vi "Set QMH Payload.vi"(8 "error in (no error)":errorcluster, 9 "Data":variant, 10 "State":enum16{""}(ring), 11 "IMessagePayload in":refnum<class "IMessagePayload.lvclass">) -> (0 "error out":errorcluster, 3 "IMessagePayload":refnum<class "IMessagePayload.lvclass">)   [LabVIEW 2016, in "QMHMessagePayload.lvclass"]
uses:
  QMHMessagePayload.lvclass
  IMessagePayload/IMessagePayload.lvclass
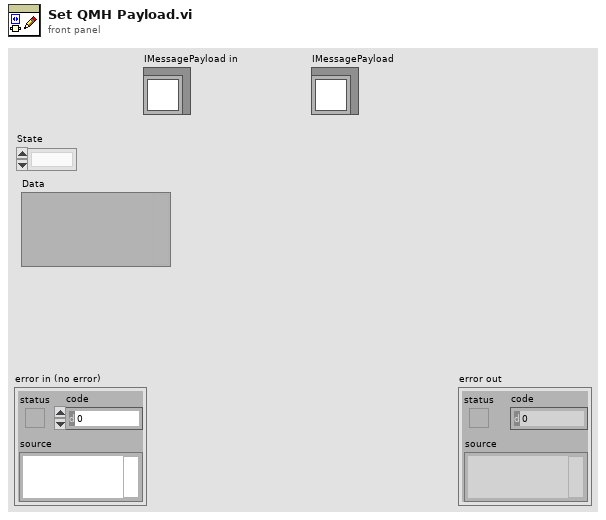
[diagram p1: front panel]
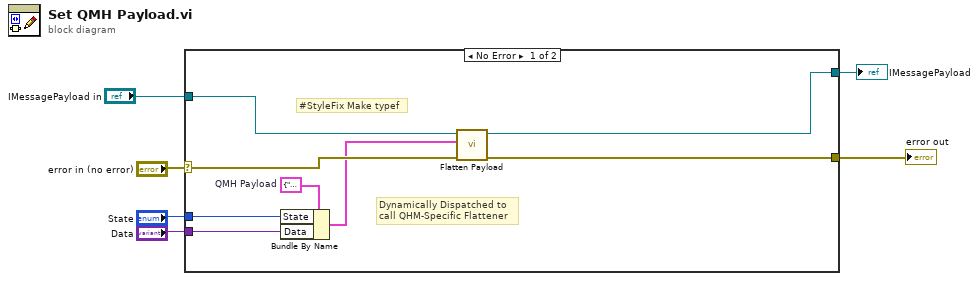
[diagram p0: block diagram]
diagram:
  n1 = case shown="No Error" "error in (no error)" {
    selector: "error in (no error)" -> [w14 w15]
    tunnel: [w13 w15] -> w5
    tunnel: "IMessagePayload in" -> [w12 _]
    tunnel: [w11 _] -> w3
    tunnel: "State" -> [w8 _]
    tunnel: "Data" -> [w7 _]
    frame No Error {
      w10 = cluster{"State":enum16{""}, "Data":variant} {"State"=enum."", "Data"=variant}  # QMH Payload
      # "#StyleFix Make typef"
      # "Dynamically Dispatched to\ncall QHM-Specific Flattener"
      n2 = Bundle By Name(cluster=w10, "State"=w8, "Data"=w7) -> (w9:cluster{"State":enum16{""}, "Data":variant})
      n3 = call-dynamic "Flatten Payload.vi"("error in (no error)"=w14, "Variant"=w9, "IMessagePayload in"=w12) -> ("error out"=w13:errorcluster, "IMessagePayload out"=w11:refnum<class "IMessagePayload.lvclass">)  [unwired: 7 in]
    }
    frame Error {
    }
  }
  "error out" <- w5
  "IMessagePayload" <- w3
